vi "PCAN_ERROR.vi"(8 "error in (no error)":errorcluster, 11 "Error Code":T1 items=["CAN_ERR_OK"=0, "CAN_ERR_XMTFULL"=1, "CAN_ERR_OVERRUN"=2, "CAN_ERR_BUSLIGHT"=4, "CAN_ERR_BUSHEAVY"=8, "CAN_ERR_BUSOFF"=16, "CAN_ERR_QRCVEMPTY"=32, "CAN_ERR_QOVERRUN"=64, "CAN_ERR_QXMTFULL"=128, "CAN_ERR_REGTEST"=256, "CAN_ERR_NOVXD"=512, "CAN_ERR_HWINUSE"=1024, "CAN_ERR_NETINUSE"=2048, "CAN_ERR_ILLHW"=5120, "CAN_ERR_ILLNET"=6144, "CAN_ERR_ILLCLINET"=7168, "CAN_ERR_RESOURCE"=8192, "CAN_ERR_ILLPARAMTYPE"=16384, "CAN_ERR_ILLPARAMVAL"=32768, "CAN_ERR_UNKNOWN"=65536]) -> (0 "error out":errorcluster, 2 "PCAN error":T2, 3 "Error Code dup":T1 items=["CAN_ERR_OK"=0, "CAN_ERR_XMTFULL"=1, "CAN_ERR_OVERRUN"=2, "CAN_ERR_BUSLIGHT"=4, "CAN_ERR_BUSHEAVY"=8, "CAN_ERR_BUSOFF"=16, "CAN_ERR_QRCVEMPTY"=32, "CAN_ERR_QOVERRUN"=64, "CAN_ERR_QXMTFULL"=128, "CAN_ERR_REGTEST"=256, "CAN_ERR_NOVXD"=512, "CAN_ERR_HWINUSE"=1024, "CAN_ERR_NETINUSE"=2048, "CAN_ERR_ILLHW"=5120, "CAN_ERR_ILLNET"=6144, "CAN_ERR_ILLCLINET"=7168, "CAN_ERR_RESOURCE"=8192, "CAN_ERR_ILLPARAMTYPE"=16384, "CAN_ERR_ILLPARAMVAL"=32768, "CAN_ERR_UNKNOWN"=65536])   [LabVIEW 2019]
uses:
  controls/PCAN_ERROR.ctl
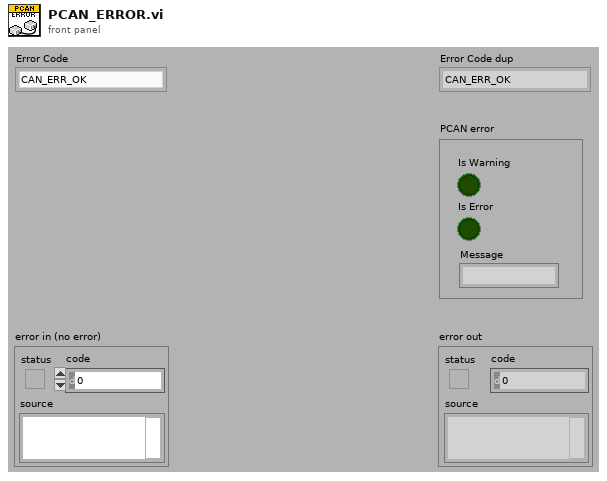
[diagram p1: front panel]
types:
  T1 = typedef "PCAN_ERROR.ctl" = i32
  T2 = cluster{"Is Warning":bool, "Is Error":bool, "Message":string}
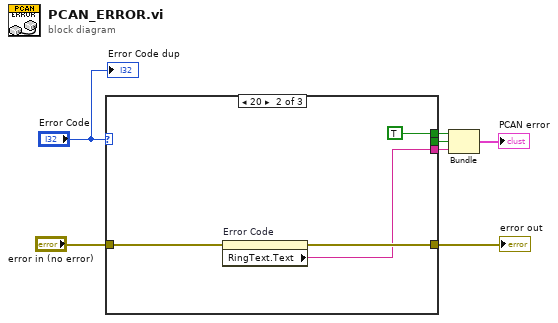
[diagram p0: block diagram]
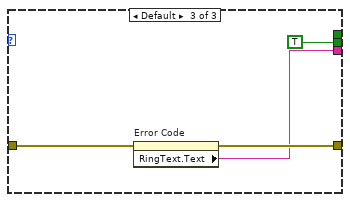
[diagram p3: hidden frame]
diagram:
  n1 = case shown="20" "Error Code" {
    tunnel: "error in (no error)" -> [w8 w11 w16]
    tunnel: [w8 w10 w15] -> w6
    tunnel: [_ w9 w14] -> w5
    tunnel: [_ _ TRUE] -> w3
    tunnel: [_ TRUE _] -> w2
    frame 0 {
    }
    frame 32 {
      n2 = property on="Error Code" class="Ring (strict)"(error in=w11) -> (error out=w10:errorcluster, "RingText.Text"=w9:string)  [unwired: 1 in, 1 out]
    }
    frame Default {
      n3 = property on="Error Code" class="Ring (strict)"(error in=w16) -> (error out=w15:errorcluster, "RingText.Text"=w14:string)  [unwired: 1 in, 1 out]
    }
  }
  "error out" <- w6
  n4 = Bundle(w2, w3, "RingText.Text"=w5) -> (→"PCAN error":cluster{bool, bool, "RingText.Text":string})  [unwired: 1 out]
  "Error Code dup" <- "Error Code"
